vi "get class data cluster.vi"(8 "error in":errorcluster, 11 "LVClassLibrary in":refnum<vi>) -> (0 "error out":errorcluster, 1 "cluster ref":refnum<vi>, 2 "class data ref":refnum<vi>, 3 "LVClassLibrary out":refnum<vi>)   [LabVIEW 2013, in "NISE Tools Scripting.lvlib"]
uses:
  NISE Tools Scripting.lvlib
  <vilib>/Utility/traverseref.llb/TRef TravTarget.ctl
  <vilib>/Utility/traverseref.llb/VI Scripting - Traverse.lvlib
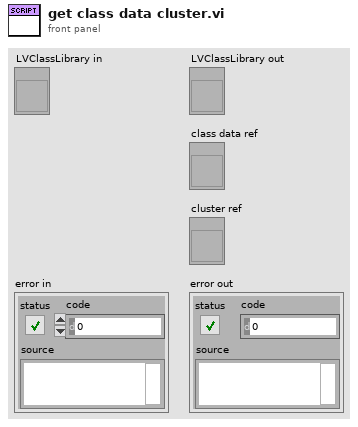
[diagram p1: front panel]
types:
  T1 = typedef "TRef TravTarget.ctl" = enum16{"FP", "BD", "Other"}
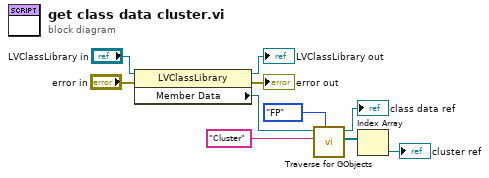
[diagram p0: block diagram]
diagram:
  n1 = property class="LVClassLibrary"(reference="LVClassLibrary in", error in="error in") -> (reference out=→"LVClassLibrary out":refnum<vi>, error out=→"error out":errorcluster, "Member Data"=w9:refnum<vi>)
  n2 = call <vilib>:"Traverse for GObjects.vi"("Traverse Target"=TRef_TravTarget."FP", "Class Name"="Cluster", "VI Refnum"=w9) -> ("References"=w8:refnum<vi>[], "dup VI Refnum"=→"class data ref":refnum<vi>)  [unwired: 5 in, 2 out]
  n3 = Index Array(array=w8) -> (element=→"cluster ref":refnum<vi>)  [unwired: 1 in]
